vi "_GetData.vi"(8 "Error In":errorcluster, 9 "Length":i32, 10 "Index Or Position":u32, 11 "ByteBuffer In":refnum<class "ByteBuffer.lvclass">) -> (0 "Error Out":errorcluster, 2 "Byte Array":u8[](array[numeric]), 3 "ByteBuffer Out":refnum<class "ByteBuffer.lvclass">)   [LabVIEW 2015, in "ByteBuffer.lvclass"]
uses:
  ByteBuffer.lvclass
  ByteBuffer.lvclass/ByteBuffer.ctl
  properties/position/Set Position.vi
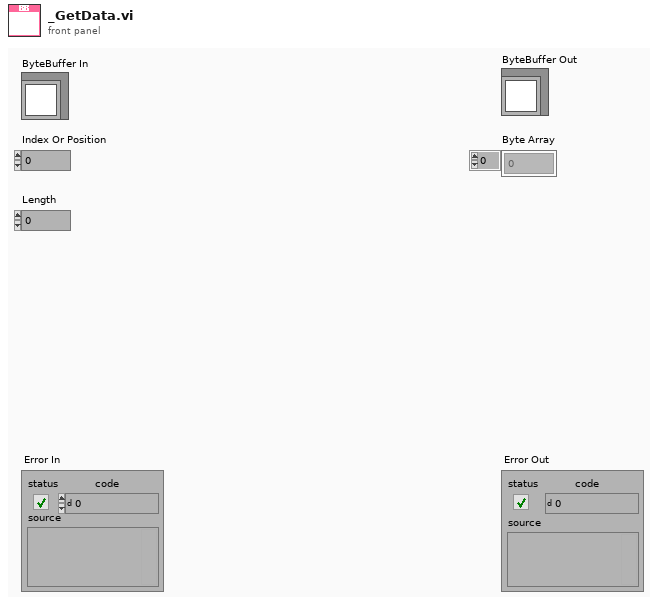
[diagram p1: front panel]
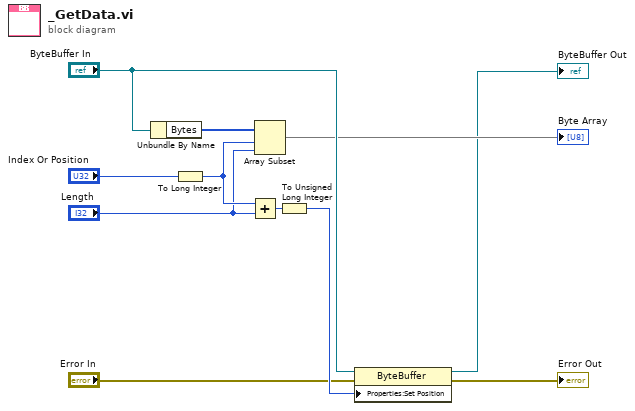
[diagram p0: block diagram]
diagram:
  n1 = Unbundle By Name("ByteBuffer In") -> ("Bytes"=w5:u8[])
  n2 = To Long Integer(number="Index Or Position") -> (32bit integer=w9:i32)
  n3 = Add(x=w9, y="Length") -> (x+y=w10:i32)
  n4 = Array Subset(array=w5, index=w9, length="Length") -> (→"Byte Array":u8[])
  n5 = To Unsigned Long Integer(number=w10) -> (unsigned 32bit integer=w7:u32)
  n6 = property class="ByteBuffer"(reference="ByteBuffer In", error in="Error In", "Properties:Set Position"=w7) -> (reference out=→"ByteBuffer Out":refnum<class "ByteBuffer.lvclass">, error out=→"Error Out":errorcluster)
